vi "NF_CALC.vi"(7 "G(db)":dbl, 8 "BW(MHz)":dbl, 10 "BandPow(dBm)":dbl) -> (3 "NF(dB)":dbl)   [LabVIEW 2018]
panel:
  # "Convert S/N to NF in DB"
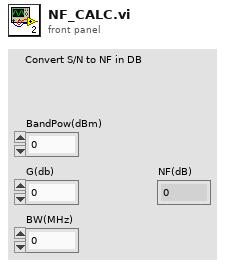
[diagram p1: front panel]
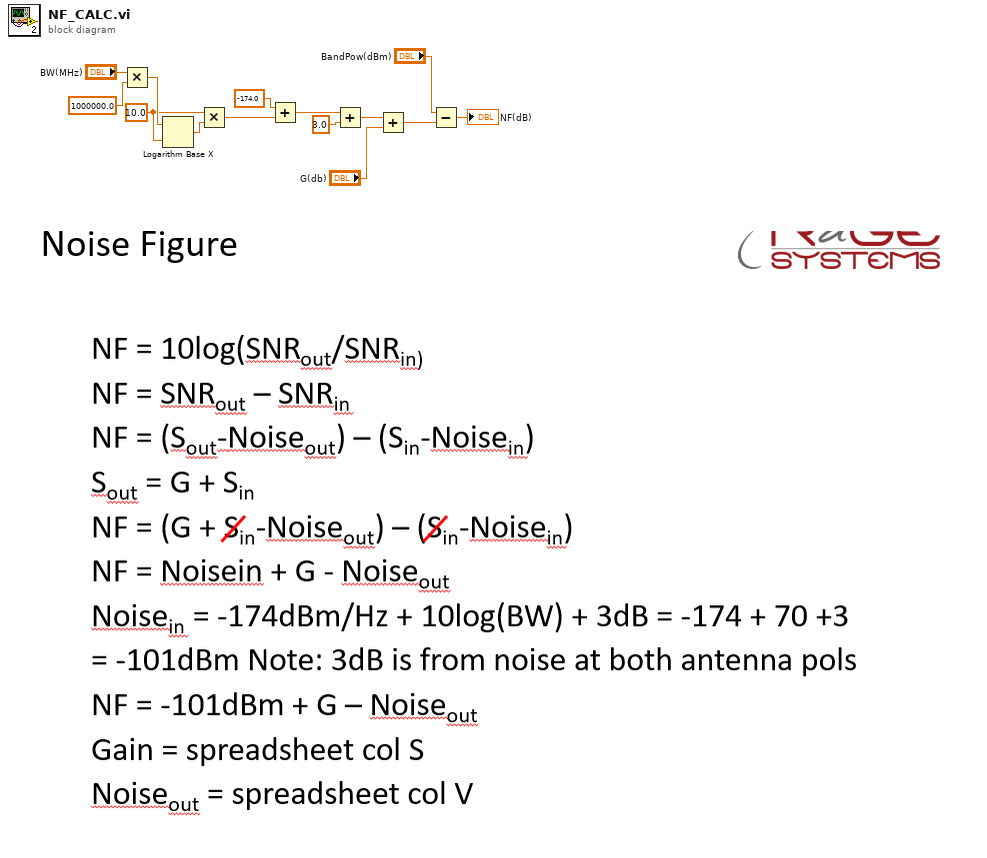
[diagram p0: block diagram]
diagram:
  w9 = 10.0 ("x")
  n1 = Multiply(x="BW(MHz)", y=1000000.0) -> (x*y=w11:dbl)
  n2 = Logarithm Base X(1:w9, 2:w11) -> (0:w10:dbl)
  n3 = Multiply(x=w9, y=w10) -> (x*y=w8:dbl)
  n4 = Add(x=-174.0, y=w8) -> (x+y=w7:dbl)
  n5 = Add(x=w7, y=3.0) -> (x+y=w3:dbl)
  n6 = Add(x=w3, y="G(db)") -> (x+y=w2:dbl)
  n7 = Subtract(x="BandPow(dBm)", y=w2) -> (x-y=→"NF(dB)":dbl)
